vi "Get World extent.vi"(0 "Triangles":T1[](array[typedef])) -> (1 "Pmax (x, y, z)":sgl[](array[numeric]), 2 "Pmin (x, y, z)":sgl[](array[numeric]))   [LabVIEW 2016]
uses:
  Typedefs/Triangle.ctl
panel:
  # "PN 18/01/2015, 08/06/2017 (pad by eps_m)"
  # "Vertices"
  # "Edges"
  # "Unit normal"
  # "Edge unit normals"
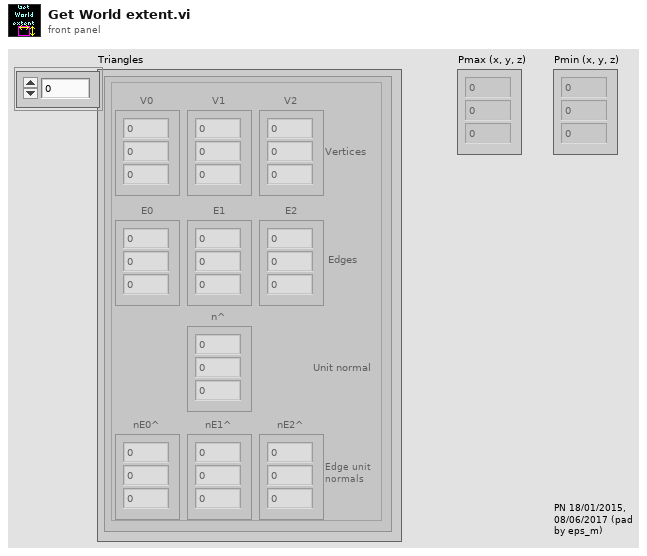
[diagram p1: front panel]
types:
  T1 = typedef "Triangle.ctl" = cluster{"V0":sgl[], "V1":sgl[], "V2":sgl[], "E0":sgl[], "E1":sgl[], "E2":sgl[], "n^":sgl[], "nE0^":sgl[], "nE1^":sgl[], "nE2^":sgl[]}
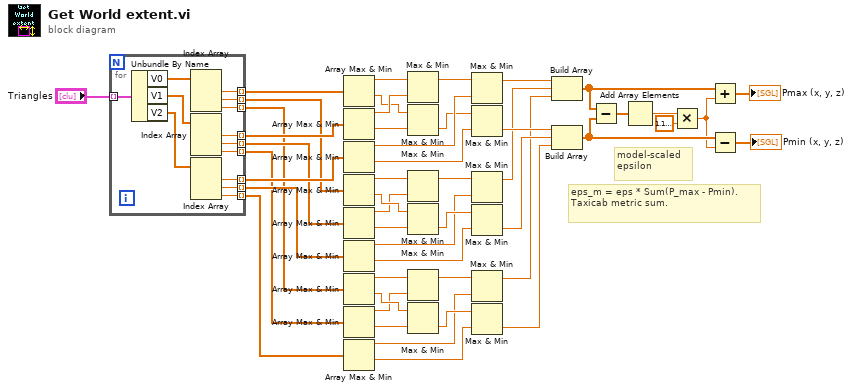
[diagram p0: block diagram]
diagram:
  # "eps_m = eps * Sum(P_max - Pmin). Taxicab metric sum."
  # "model-scaled epsilon"
  n1 = for {
    tunnel: "Triangles" -> [w61] mode=indexing
    tunnel: [w57] -> w47 mode=indexing
    tunnel: [w56] -> w44 mode=indexing
    tunnel: [w55] -> w41 mode=indexing
    tunnel: [w54] -> w46 mode=indexing
    tunnel: [w53] -> w43 mode=indexing
    tunnel: [w52] -> w40 mode=indexing
    tunnel: [w51] -> w45 mode=indexing
    tunnel: [w50] -> w42 mode=indexing
    tunnel: [w49] -> w39 mode=indexing
    n2 = Unbundle By Name(w61) -> ("V0"=w60:sgl[], "V1"=w59:sgl[], "V2"=w58:sgl[])
    n3 = Index Array(array=w60) -> (element #1=w57:sgl, element #2=w56:sgl, element #3=w55:sgl)  [unwired: 3 in]
    n4 = Index Array(array=w59) -> (element #1=w54:sgl, element #2=w53:sgl, element #3=w52:sgl)  [unwired: 3 in]
    n5 = Index Array(array=w58) -> (element #1=w51:sgl, element #2=w50:sgl, element #3=w49:sgl)  [unwired: 3 in]
  }
  n6 = Array Max & Min(array=w47) -> (max value=w38:sgl, min value=w33:sgl)  [unwired: 2 out]
  n7 = Array Max & Min(array=w46) -> (max value=w37:sgl, min value=w32:sgl)  [unwired: 2 out]
  n8 = Array Max & Min(array=w45) -> (max value=w35:sgl, min value=w30:sgl)  [unwired: 2 out]
  n9 = Array Max & Min(array=w44) -> (max value=w26:sgl, min value=w25:sgl)  [unwired: 2 out]
  n10 = Array Max & Min(array=w43) -> (max value=w24:sgl, min value=w23:sgl)  [unwired: 2 out]
  n11 = Array Max & Min(array=w42) -> (max value=w22:sgl, min value=w21:sgl)  [unwired: 2 out]
  n12 = Array Max & Min(array=w41) -> (max value=w16:sgl, min value=w15:sgl)  [unwired: 2 out]
  n13 = Array Max & Min(array=w40) -> (max value=w14:sgl, min value=w13:sgl)  [unwired: 2 out]
  n14 = Array Max & Min(array=w39) -> (max value=w12:sgl, min value=w11:sgl)  [unwired: 2 out]
  n15 = Max & Min(x=w38, y=w37) -> (max(x,y)=w36:sgl)  [unwired: 1 out]
  n16 = Max & Min(x=w33, y=w32) -> (min(x,y)=w31:sgl)  [unwired: 1 out]
  n17 = Max & Min(x=w26, y=w24) -> (max(x,y)=w27:sgl)  [unwired: 1 out]
  n18 = Max & Min(x=w25, y=w23) -> (min(x,y)=w28:sgl)  [unwired: 1 out]
  n19 = Max & Min(x=w16, y=w14) -> (max(x,y)=w18:sgl)  [unwired: 1 out]
  n20 = Max & Min(x=w15, y=w13) -> (min(x,y)=w17:sgl)  [unwired: 1 out]
  n21 = Max & Min(x=w36, y=w35) -> (max(x,y)=w34:sgl)  [unwired: 1 out]
  n22 = Max & Min(x=w31, y=w30) -> (min(x,y)=w29:sgl)  [unwired: 1 out]
  n23 = Max & Min(x=w27, y=w22) -> (max(x,y)=w20:sgl)  [unwired: 1 out]
  n24 = Max & Min(x=w28, y=w21) -> (min(x,y)=w19:sgl)  [unwired: 1 out]
  n25 = Max & Min(x=w18, y=w12) -> (max(x,y)=w10:sgl)  [unwired: 1 out]
  n26 = Max & Min(x=w17, y=w11) -> (min(x,y)=w9:sgl)  [unwired: 1 out]
  n27 = Build Array(w34, w20, w10) -> (w6:sgl[])
  n28 = Build Array(w29, w19, w9) -> (w5:sgl[])
  n29 = Subtract(x=w6, y=w5) -> (x-y=w4:sgl[])
  n30 = Add Array Elements(numeric array=w4) -> (sum=w3:sgl)
  n31 = Multiply(x=w3, y=sgl 1.1920929e-07) -> (x*y=w1:sgl)
  n32 = Add(x=w6, y=w1) -> (x+y=→"Pmax (x, y, z)":sgl[])
  n33 = Subtract(x=w5, y=w1) -> (x-y=→"Pmin (x, y, z)":sgl[])
